vi "SubVI_ErrorChecking_Ger_Funcoes.vi"(0 "Gerador de Funções":refnum<visa-resource-name>="GPIB0::10::INSTR") -> (1 "VISA resource name out":refnum<visa-resource-name>, 2 "ERROR":bool)   [LabVIEW 2018]
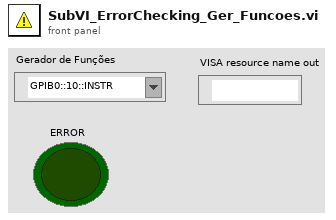
[diagram p1: front panel]
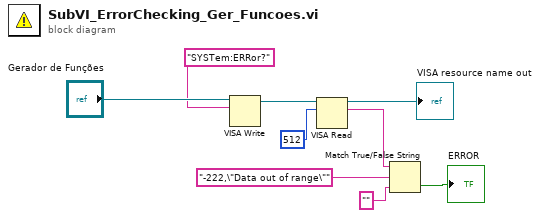
[diagram p0: block diagram]
diagram:
  n1 = VISA Write(VISA resource name="Gerador de Funções", write buffer="SYSTem:ERRor?") -> (VISA resource name out=w7:refnum<visa-resource-name>)  [unwired: 1 in, 2 out]
  n2 = VISA Read(VISA resource name=w7, byte count=u32 512) -> (VISA resource name out=→"VISA resource name out":refnum<visa-resource-name>, read buffer=w1:string)  [unwired: 1 in, 2 out]
  n3 = Match True/False String(2:"" ("false string"), 3:"-222,\"Data out of range\"" ("true string"), 4:w1) -> (0:→"ERROR":bool)  [unwired: 1 out]
